vi "HGF_ImaqFg.appendData2Variant.vi"(0 "initData":variant, 5 "error in (no error)":errorcluster) -> (14 "dup initData":variant, 19 "error out":errorcluster)   [LabVIEW 2014, in "HGF_IMAQ.lvlib" / "HGF_ImaqFg.lvclass"]
uses:
  HGF_ImaqFg.lvclass
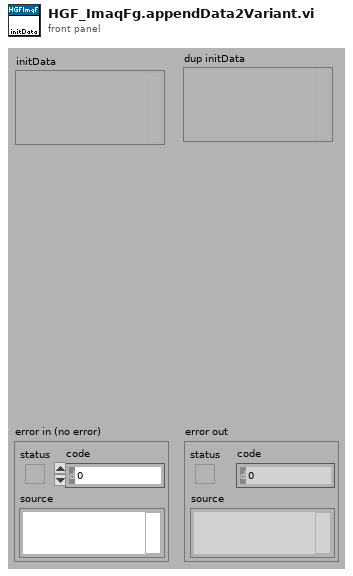
[diagram p1: front panel]
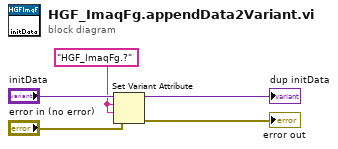
[diagram p0: block diagram]
diagram:
  w1 = "HGF_ImaqFg.?" ("name")
  n1 = Set Variant Attribute(Variant="initData", name=w1, value=w1, error in="error in (no error)") -> (Variant out=→"dup initData":variant, error out=→"error out":errorcluster)  [unwired: 1 out]
